vi "Waveform Scan Done.vi"(8 "error in (no error)":errorcluster, 11 "Model in":refnum<class "Model.lvclass">) -> (0 "error out":errorcluster, 2 "Done":bool, 3 "Model out":refnum<class "Model.lvclass">)   [LabVIEW 2015, in "Model.lvclass"]
uses:
  Model.lvclass
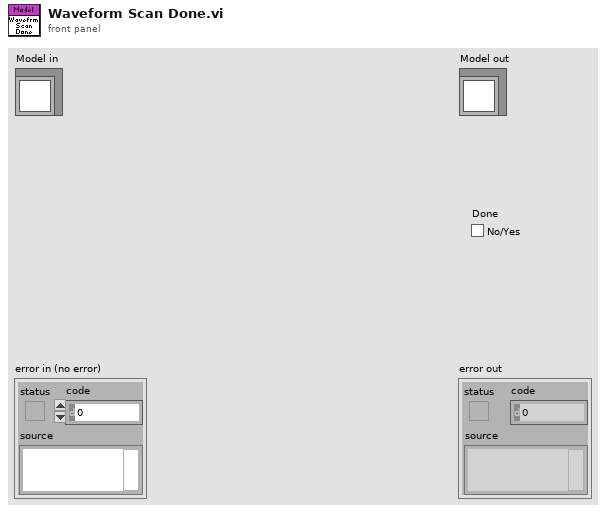
[diagram p1: front panel]
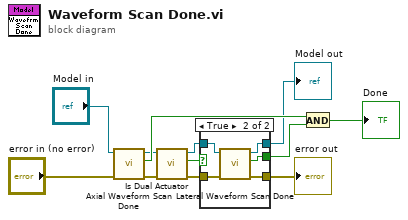
[diagram p0: block diagram]
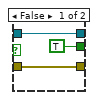
[diagram p2: hidden frame]
diagram:
  n1 = call "Axial Waveform Scan Done.vi"("error in (no error)"="error in (no error)", "Model in"="Model in") -> ("error out"=w5:errorcluster, "Done"=w11:bool, "Model out"=w1:refnum<class "Model.lvclass">)  [unwired: 7 in]
  n2 = call "Is Dual Actuator.vi"("error in (no error)"=w5, "Model in"=w1) -> ("error out"=w4:errorcluster, "Is Dual Actuator"=w3:bool, "Model out"=w2:refnum<class "Model.lvclass">)  [unwired: 7 in]
  n3 = case shown="True" w3 {
    tunnel: [TRUE ("Done") w20] -> w12
    tunnel: [w14 w19] -> w9
    tunnel: w2 -> [w14 w18]
    tunnel: w4 -> [w13 w17]
    tunnel: [w13 w16] -> w6
    frame False {
    }
    frame True {
      n4 = call "Lateral Waveform Scan Done.vi"("error in (no error)"=w17, "Model in"=w18) -> ("error out"=w16:errorcluster, "Done"=w20:bool, "Model out"=w19:refnum<class "Model.lvclass">)  [unwired: 7 in]
    }
  }
  "error out" <- w6
  "Model out" <- w9
  n5 = And(x=w11, y=w12) -> (x .and. y?=→"Done":bool)
